vi "SystemGetScreenImage.vi"(8 "error in (no error)":errorcluster {"code" format="%.0x"}, 9 "ImageBufferSize":i32=2048 caption="ImageBufferSize (2048)", 11 "instrument handle":refnum<k15>) -> (0 "error out":errorcluster {"code" format="%.0x"}, 1 "ImageActualSize":i32, 2 "Image":u8[](array[numeric]), 3 "instrument handle out":refnum<k15>)   [LabVIEW 2009, in "Keysight XSAn.lvlib"]
doc: "Retuns an array whose contents may be saved as a GIF image file (.gif) of the current display.\n\nSupported Models: All supported"
uses:
  <instrlib>/Keysight XSAn/Keysight XSAn.lvlib
  AgXSAn.dll
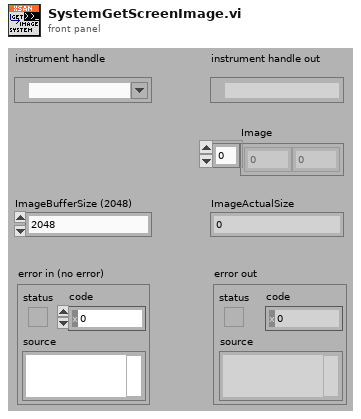
[diagram p1: front panel]
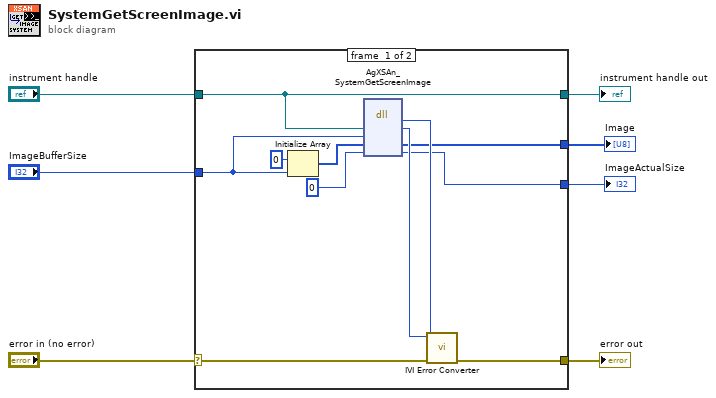
[diagram p0: block diagram]
diagram:
  n1 = case shown="No Error" "error in (no error)" {
    selector: "error in (no error)" -> [w16 w20]
    tunnel: [w15 w20] -> w7
    tunnel: "instrument handle" -> [w10 w19]
    tunnel: "ImageBufferSize" -> [w9 _]
    tunnel: [w13 _] -> w3
    tunnel: [w11 _] -> w2
    tunnel: [w10 w19] -> w1
    frame #0 {
      n2 = Initialize Array(u8 0 ("element"), w9) -> (w8:u8[])
      n3 = dll-call lib="AgXSAn**.dll" fn="AgXSAn_SystemGetScreenImage"("Vi"=w10, "ImageBufferSize"=w9, "Image"=w8, "ImageActualSize"=0) -> ("return type"=w17:i32, "Vi"=w18:u32, "Image"=w13:u8[], "ImageActualSize"=w11:i32)  [unwired: 4 in, 2 out]
      n4 = call <instrlib>:"IVI Error Converter.vi"("error in (no error)"=w16, "IVI error code (0)"=w17, "instrument handle"=w18) -> ("error out"=w15:errorcluster)  [unwired: 7 in, 1 out]
    }
    frame #1 {
    }
  }
  "error out" <- w7
  "instrument handle out" <- w1
  "Image" <- w3
  "ImageActualSize" <- w2
